vi "zang-suen_Sub.vi"(9 "Numerisch (Eingang)":i32, 10 "Modus":enum16{"thinning", "skeleton"}(ring), 11 "Template":bool[][](array[boolean])) -> (2 "Numerisch (Ausgang)":i32, 3 "Array":bool[][](array[boolean]))   [LabVIEW 2017]
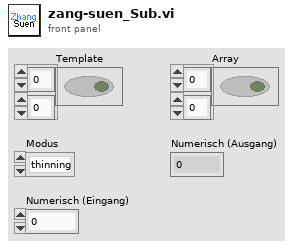
[diagram p1: front panel]
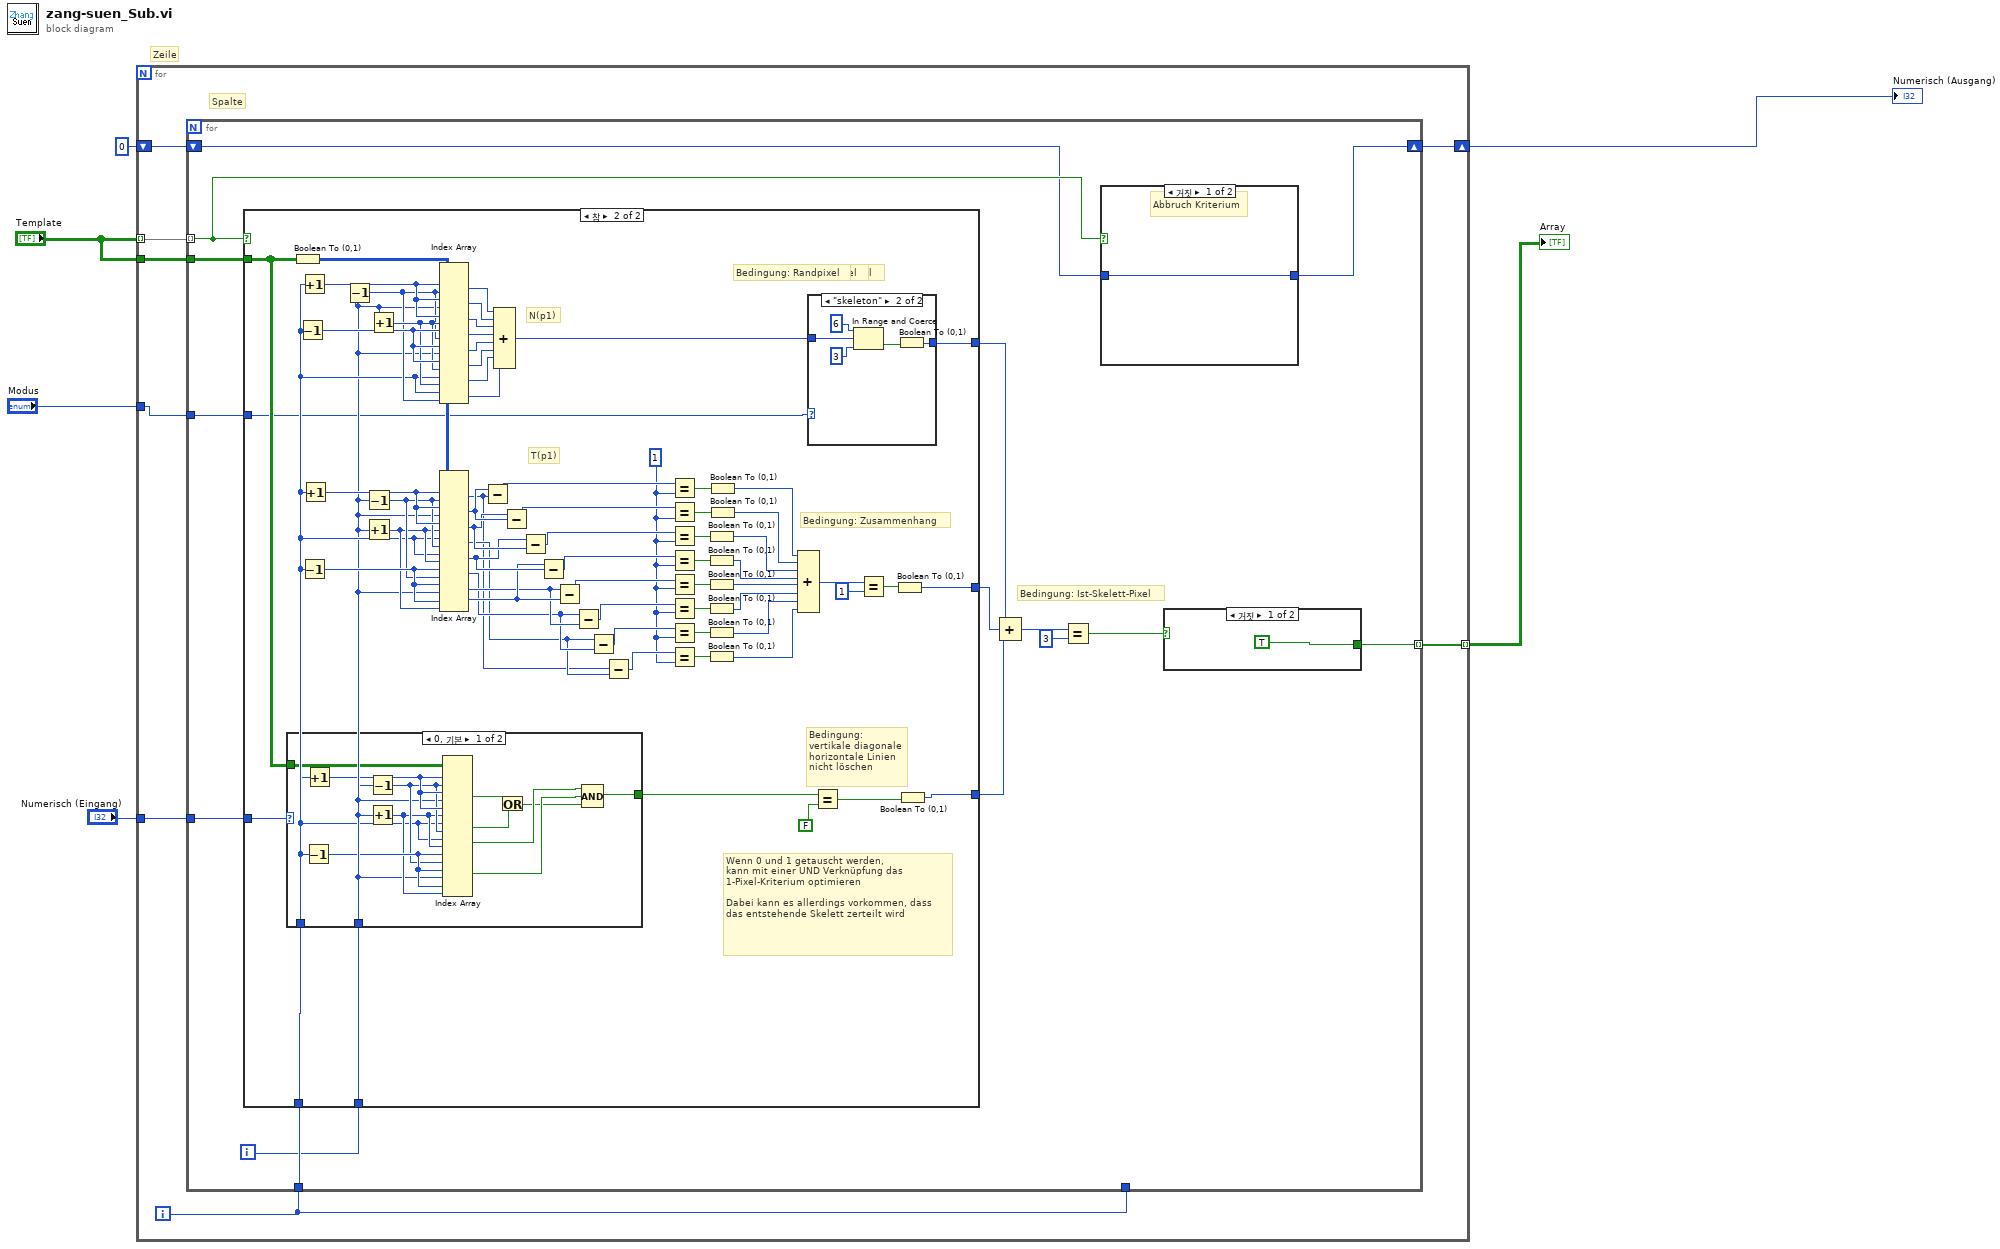
[diagram p0: block diagram]
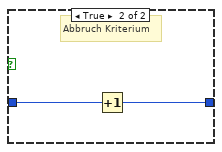
[diagram p2: hidden frame]
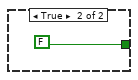
[diagram p3: hidden frame]
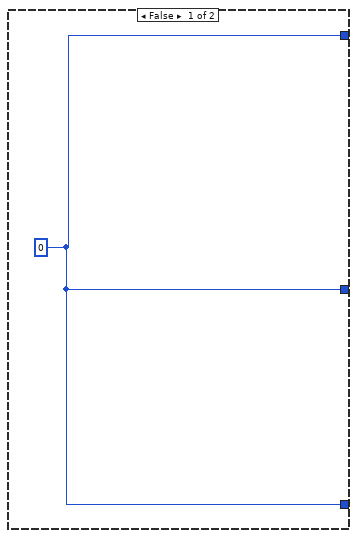
[diagram p4: hidden frame]
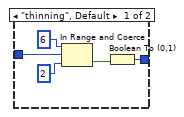
[diagram p5: hidden frame]
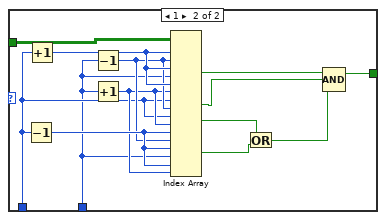
[diagram p6: hidden frame]
diagram:
  # "Zeile"
  n1 = for {
    tunnel: "Template" -> [w14] mode=indexing
    tunnel: "Template" -> [w13]
    tunnel: [w11] -> w2 mode=indexing
    tunnel: "Numerisch (Eingang)" -> [w10]
    shift-right: [w9] -> w5
    shift-left: 0 -> [w8]
    tunnel: "Modus" -> [w7]
    i -> [w12]
    # "Spalte"
    n2 = for {
      tunnel: w14 -> [w18] mode=indexing
      tunnel: w13 -> [w24]
      tunnel: w12 -> [w29]
      tunnel: w12 -> [_]
      tunnel: [w21] -> w11 mode=indexing
      tunnel: w10 -> [w20]
      shift-right: [w16] -> w9
      shift-left: w8 -> [w17]
      tunnel: w7 -> [w15]
      i -> [w23]
      # "Bedingung: Ist-Skelett-Pixel"
      n3 = case shown="참" w18 {
        tunnel: w24 -> [_ w40]
        tunnel: w23 -> [_ w43]
        tunnel: w29 -> [_ w44]
        tunnel: [w35 w50] -> w27
        tunnel: [w35 w46] -> w28
        tunnel: [w35 w42] -> w19
        tunnel: w20 -> [_ w41]
        tunnel: w15 -> [_ w36]
        frame False {
          w35 = 0
        }
        frame True {
          w67 = 1
          # "Wenn 0 und 1 getauscht werden,\nkann mit einer UND Verknüpfung das \n1-Pixel-Kriterium optimieren\n\nDabei kann es allerdings vorkommen, dass \ndas entstehende Skelett zerteilt wird"
          # "Mehr als ein nicht Randpixel"
          # "Bedingung:\nvertikale diagonale\nhorizontale Linien\nnicht löschen"
          # "Bedingung: Zusammenhang"
          # "Bedingung: kein Endpixel"
          # "Bedingung: Randpixel"
          # "T(p1)"
          # "N(p1)"
          n4 = case shown="0, 기본" w41 {
            tunnel: w40 -> [w119 w132]
            tunnel: w44 -> [w118 w131]
            tunnel: w43 -> [w117 w130]
            tunnel: [w116 w124] -> w38
            frame 0, Default {
              n5 = Decrement(x=w118) -> (x-1=w122:i32)
              n6 = Increment(x=w118) -> (x+1=w123:i32)
              n7 = Decrement(x=w117) -> (x-1=w121:i32)
              n8 = Increment(x=w117) -> (x+1=w120:i32)
              n9 = Index Array(array=w119, index (row) #1=w123, index (col) #1=w121, index (row) #2=w123, index (col) #2=w117, index (row) #3=w123, index (col) #3=w120, index (row) #4=w118, index (col) #4=w121, index (row) #5=w118, index (col) #5=w120, index (row) #6=w122, index (col) #6=w121, index (row) #7=w122, index (col) #7=w117, index (row) #8=w122, index (col) #8=w120) -> (element #2=w112:bool, element #4=w113:bool, element #5=w115:bool, element #7=w114:bool)  [unwired: 4 out]
              n10 = Or(x=w112, y=w113) -> (x .or. y?=w111:bool)
              n11 = Compound Arithmetic op=AND(w115, w114, w111) -> (w116:bool)
            }
            frame 1 {
              n12 = Decrement(x=w131) -> (x-1=w135:i32)
              n13 = Increment(x=w131) -> (x+1=w136:i32)
              n14 = Decrement(x=w130) -> (x-1=w134:i32)
              n15 = Increment(x=w130) -> (x+1=w133:i32)
              n16 = Index Array(array=w132, index (row) #1=w136, index (col) #1=w134, index (row) #2=w136, index (col) #2=w130, index (row) #3=w136, index (col) #3=w133, index (row) #4=w131, index (col) #4=w134, index (row) #5=w131, index (col) #5=w133, index (row) #6=w135, index (col) #6=w134, index (row) #7=w135, index (col) #7=w130, index (row) #8=w135, index (col) #8=w133) -> (element #2=w129:bool, element #4=w128:bool, element #5=w126:bool, element #7=w127:bool)  [unwired: 4 out]
              n17 = Or(x=w126, y=w127) -> (x .or. y?=w125:bool)
              n18 = Compound Arithmetic op=AND(w129, w128, w125) -> (w124:bool)
            }
          }
          n19 = Boolean To (0,1)(Boolean=w40) -> (0, 1=w45:i16[][])
          n20 = Decrement(x=w44) -> (x-1=w99:i32)
          n21 = Increment(x=w44) -> (x+1=w100:i32)
          n22 = Decrement(x=w44) -> (x-1=w86:i32)
          n23 = Increment(x=w44) -> (x+1=w87:i32)
          n24 = Decrement(x=w43) -> (x-1=w97:i32)
          n25 = Decrement(x=w43) -> (x-1=w85:i32)
          n26 = Increment(x=w43) -> (x+1=w84:i32)
          n27 = Increment(x=w43) -> (x+1=w98:i32)
          n28 = Index Array(array=w45, index (row) #1=w100, index (col) #1=w97, index (row) #2=w100, index (col) #2=w43, index (row) #3=w100, index (col) #3=w98, index (row) #4=w99, index (col) #4=w97, index (row) #5=w99, index (col) #5=w43, index (row) #6=w99, index (col) #6=w98, index (row) #7=w44, index (col) #7=w98, index (row) #8=w44, index (col) #8=w97) -> (element #1=w96:i16, element #2=w95:i16, element #3=w94:i16, element #4=w93:i16, element #5=w92:i16, element #6=w91:i16, element #7=w90:i16, element #8=w89:i16)
          n29 = Index Array(array=w45, index (row) #1=w87, index (col) #1=w85, index (row) #2=w87, index (col) #2=w43, index (row) #3=w87, index (col) #3=w84, index (row) #4=w44, index (col) #4=w85, index (row) #5=w44, index (col) #5=w84, index (row) #6=w86, index (col) #6=w85, index (row) #7=w86, index (col) #7=w43, index (row) #8=w86, index (col) #8=w84) -> (element #1=w76:i16, element #2=w83:i16, element #3=w82:i16, element #4=w77:i16, element #5=w81:i16, element #6=w78:i16, element #7=w79:i16, element #8=w80:i16)
          n30 = Subtract(x=w83, y=w76) -> (x-y=w75:i16)
          n31 = Compound Arithmetic op=ADD(w96, w95, w94, w93, w92, w91, w90, w89) -> (w88:i16)
          n32 = Subtract(x=w82, y=w83) -> (x-y=w74:i16)
          n33 = Subtract(x=w81, y=w82) -> (x-y=w73:i16)
          n34 = Subtract(x=w80, y=w81) -> (x-y=w72:i16)
          n35 = Subtract(x=w79, y=w80) -> (x-y=w71:i16)
          n36 = Subtract(x=w78, y=w79) -> (x-y=w70:i16)
          n37 = Subtract(x=w77, y=w78) -> (x-y=w69:i16)
          n38 = Subtract(x=w76, y=w77) -> (x-y=w68:i16)
          n39 = Equal?(x=w75, y=w67) -> (x = y?=w66:bool)
          n40 = Equal?(x=w74, y=w67) -> (x = y?=w65:bool)
          n41 = Equal?(x=w73, y=w67) -> (x = y?=w64:bool)
          n42 = Equal?(x=w72, y=w67) -> (x = y?=w63:bool)
          n43 = Equal?(x=w71, y=w67) -> (x = y?=w62:bool)
          n44 = Equal?(x=w70, y=w67) -> (x = y?=w61:bool)
          n45 = Equal?(x=w69, y=w67) -> (x = y?=w60:bool)
          n46 = Equal?(x=w68, y=w67) -> (x = y?=w59:bool)
          n47 = Boolean To (0,1)(Boolean=w64) -> (0, 1=w56:i16)
          n48 = Boolean To (0,1)(Boolean=w63) -> (0, 1=w55:i16)
          n49 = Boolean To (0,1)(Boolean=w62) -> (0, 1=w54:i16)
          n50 = Boolean To (0,1)(Boolean=w61) -> (0, 1=w53:i16)
          n51 = Boolean To (0,1)(Boolean=w60) -> (0, 1=w52:i16)
          n52 = Boolean To (0,1)(Boolean=w59) -> (0, 1=w51:i16)
          n53 = Boolean To (0,1)(Boolean=w66) -> (0, 1=w58:i16)
          n54 = Boolean To (0,1)(Boolean=w65) -> (0, 1=w57:i16)
          n55 = Compound Arithmetic op=ADD(w58, w57, w56, w55, w54, w53, w52, w51) -> (w49:i16)
          n56 = case shown="\"skeleton\"" w36 {
            tunnel: w88 -> [w103 w108]
            tunnel: [w101 w106] -> w50
            frame "thinning", Default {
              n57 = In Range and Coerce(upper limit=6 ("Obergrenze"), x=w103, lower limit=2 ("Untergrenze")) -> (In Range?=w102:bool)  [unwired: 1 out]
              n58 = Boolean To (0,1)(Boolean=w102) -> (0, 1=w101:i16)
            }
            frame "skeleton" {
              n59 = In Range and Coerce(upper limit=6 ("Obergrenze"), x=w108, lower limit=3 ("Untergrenze")) -> (In Range?=w107:bool)  [unwired: 1 out]
              n60 = Boolean To (0,1)(Boolean=w107) -> (0, 1=w106:i16)
            }
          }
          n61 = Equal?(x=w38, y=FALSE) -> (x = y?=w37:bool)
          n62 = Equal?(x=w49, y=i16 1) -> (x = y?=w47:bool)
          n63 = Boolean To (0,1)(Boolean=w47) -> (0, 1=w46:i16)
          n64 = Boolean To (0,1)(Boolean=w37) -> (0, 1=w42:i16)
        }
      }
      n65 = Compound Arithmetic op=ADD(w27, w28, w19) -> (w26:i32)
      n66 = Equal?(x=w26, y=3) -> (x = y?=w22:bool)
      n67 = case shown="거짓" w18 {
        tunnel: w17 -> [w30 w32]
        tunnel: [w30 w31] -> w16
        frame False {
          # "Abbruch Kriterium"
        }
        frame True {
          # "Abbruch Kriterium"
          n68 = Increment(x=w32) -> (x+1=w31:i32)
        }
      }
      n69 = case shown="거짓" w22 {
        tunnel: [TRUE FALSE] -> w21
        frame False {
        }
        frame True {
        }
      }
    }
  }
  "Numerisch (Ausgang)" <- w5
  "Array" <- w2
